vi "2401 Wire.vi"(9 "4-wire":bool) -> ()   [LabVIEW 2011]
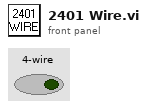
[diagram p1: front panel]
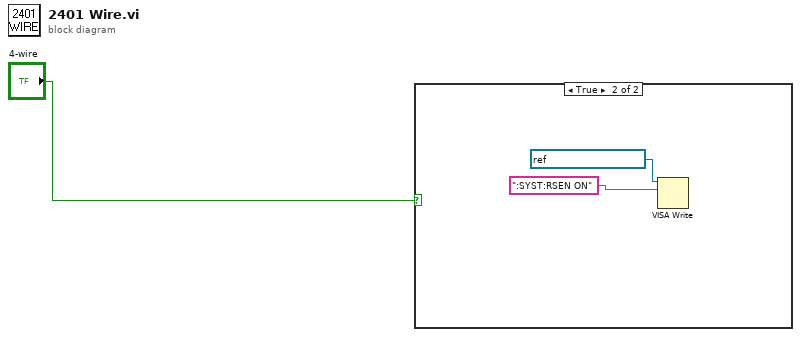
[diagram p0: block diagram]
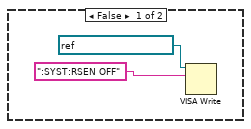
[diagram p2: hidden frame]
diagram:
  n1 = case shown="True" "4-wire" {
    frame False {
      n2 = VISA Write(VISA resource name=refnum<visa-resource-name> "GPIB0::13::INSTR", write buffer=":SYST:RSEN OFF") -> ()  [unwired: 1 in, 3 out]
    }
    frame True {
      n3 = VISA Write(VISA resource name=refnum<visa-resource-name> "GPIB0::13::INSTR", write buffer=":SYST:RSEN ON") -> ()  [unwired: 1 in, 3 out]
    }
  }
